vi "Write Handler Output Data.vi"(8 "error in (no error)":errorcluster, 9 "Data (1)":i32=1, 10 "Port (0: A)":u16(ring) items=["A", "B", "C", "D", "E", "F", "G", "H"], 11 "VISA resource name":refnum<visa-resource-name>) -> (0 "error out":errorcluster, 3 "VISA resource name out":refnum<visa-resource-name>)   [LabVIEW 2022 SP3, in "Agilent ENA Series.lvlib"]
doc: "Outputs data to output port A (A0 to A7), port B (B0 to B7), port C (C0 to C3), port D (D0 to D3), port E (C0 to D3) or port F (A0 to B7).\n\nNotes:\n(1) Ports C or D must be set to output mode for set to the port C or D.\n(2) Ports C and D must be set to output mode for set to the port E.\n(3) Data is outputted as 8-bit binary (for port A and B) using x0 as LSB and x7 as MSB. Where x is port name.\n(4) Data is outputted as 4-bit binary (for port C and D) using x0 as LSB and x3 as MSB. Where x is port name.\n(5) Data is outputted as 8-bit binary (for port E) using C0 as LSB and D3 as MSB.\n(6) Data is outputted as 16-bit binary (for port F) using A0 as LSB and B7 as MSB."
uses:
  <instrlib>/Agilent ENA Series/Agilent ENA Series.lvlib
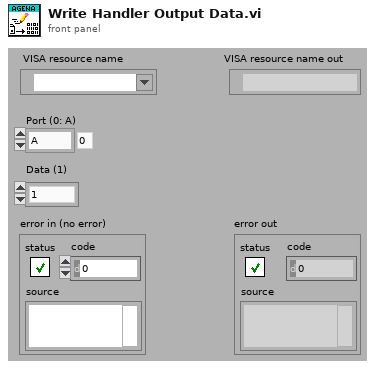
[diagram p1: front panel]
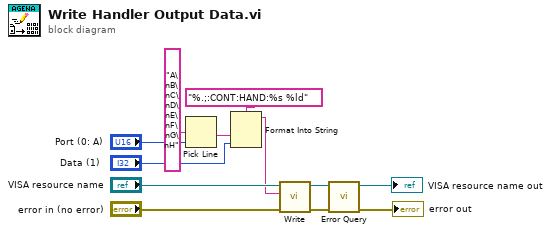
[diagram p0: block diagram]
diagram:
  n1 = Pick Line(multi-line string="A\nB\nC\nD\nE\nF\nG\nH", line index="Port (0: A)") -> (output string=w6:string)  [unwired: 1 in]
  n2 = Format Into String(format string="%.;:CONT:HAND:%s %ld", w6, "Data (1)") -> (resulting string=w9:string)  [unwired: 2 in, 1 out]
  n3 = call <instrlib>:"Write.vi"("error in (no error)"="error in (no error)", "String ()"=w9, "VISA resource name"="VISA resource name") -> ("error out"=w3:errorcluster, "VISA resource name out"=w4:refnum<visa-resource-name>)  [unwired: 6 in, 1 out]
  n4 = call <instrlib>:"Error Query.vi"("error in (no error)"=w3, "VISA resource name"=w4) -> ("error out"=→"error out":errorcluster, "VISA resource name out"=→"VISA resource name out":refnum<visa-resource-name>)  [unwired: 6 in, 2 out]
